vi "Ctor.vi"(8 "error in (no error)":errorcluster, 11 "WebProjectPanel in":refnum<class "WebProjectPanel.lvclass">) -> (0 "error out":errorcluster, 3 "WebProjectPanel out":refnum<class "WebProjectPanel.lvclass">)   [LabVIEW 2020, in "PicoG-Processor.lvlib" / "WebProjectPanel.lvclass"]
uses:
  WebProjectPanel.lvclass
  Ref Data.ctl
  WebProjectPanel.lvclass/WebProjectPanel.ctl
  <vilib>/IlluminatedG/IG OOPanel/OOPanel/ArrayPanel/ArrayPanel.lvclass
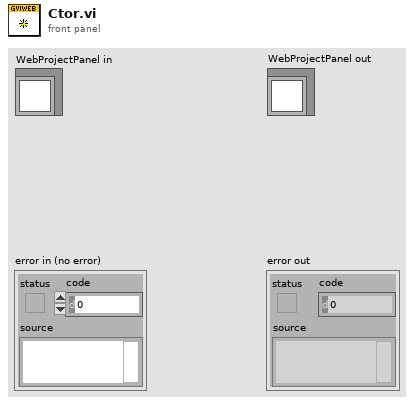
[diagram p1: front panel]
types:
  T1 = typedef "PicoG-Processor.lvlib/WebProjectPanel.lvclass/Ref Data.ctl" = cluster{"Last Update":dbl, "Path":path, "App Name":string, "Build Present":bool, "Deploy":refnum<user-event>}
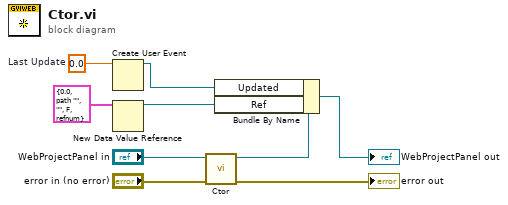
[diagram p0: block diagram]
diagram:
  w2 = 0.0  # Last Update
  n1 = Create User Event(user event datatype=w2) -> (user event=w1:refnum<user-event>)  [unwired: 1 in, 1 out]
  n2 = New Data Value Reference(data value=T1 {"Last Update"=0.0, "Path"=path "", "App Name"="", "Build Present"=FALSE, "Deploy"=refnum} ("Ref Data")) -> (data value reference=w6:refnum<data-value>)  [unwired: 1 in, 1 out]
  n3 = call-parent "Ctor.vi"("error in (no error)"="error in (no error)", "ArrayPanel in"="WebProjectPanel in") -> ("error out"=→"error out":errorcluster, "ArrayPanel out"=w5:refnum<class "WebProjectPanel.lvclass">)  [unwired: 8 in]
  n4 = Bundle By Name(cluster=w5, "Updated"=w1, "Ref"=w6) -> (→"WebProjectPanel out":refnum<class "WebProjectPanel.lvclass">)
